vi "OuputMixer5782_1Ghz_interpolated.vi"(8 "input valid":bool=TRUE, 9 "Sine in":fxp<+/-,16,0>[](array[numeric])=[0.0, 0.0, 0.0, 0.0, 0.0, 0.0, 0.0, 0.0], 10 "Cosine in":fxp<+/-,16,0>[](array[numeric])=[0.0, 0.0, 0.0, 0.0, 0.0, 0.0, 0.0, 0.0], 11 "Data":fxp<+/-,16,14>[](array[numeric])=[0.0, 0.0]) -> (3 "test":i16[](array[numeric]))   [LabVIEW 2013]
doc: "Outputs input from channel 0 as I*cos(t)-Q*sin(t) on analog output 0"
uses:
  <vilib>/rvi/eio/common/nirviEmuTemplateMethod_errors.vi
  <vilib>/eio/EIONode/EIONode.xnode
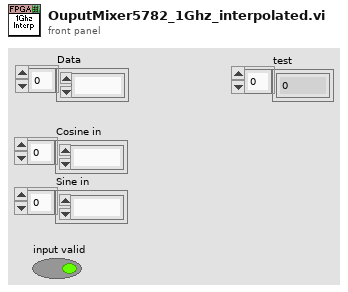
[diagram p1: front panel]
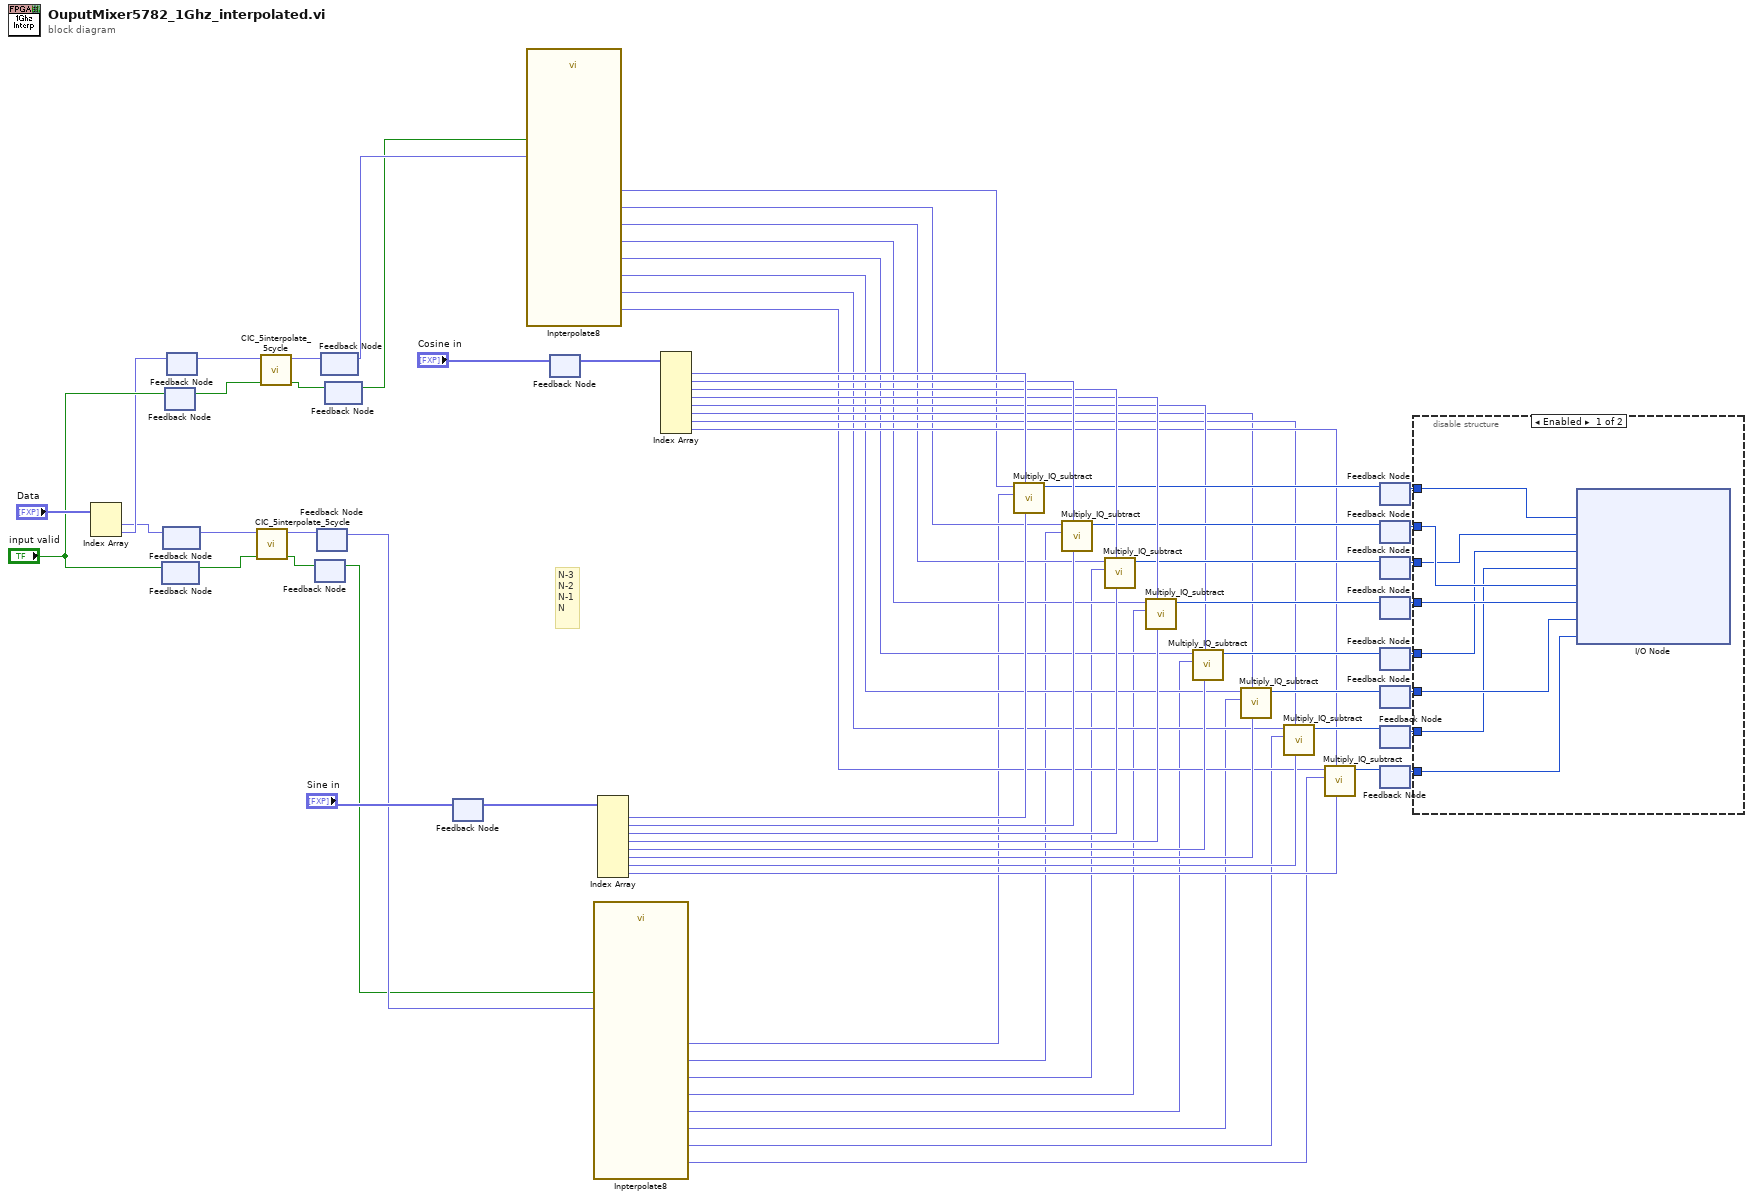
[diagram p0: block diagram]
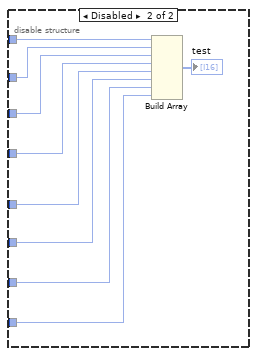
[diagram p2: hidden frame]
diagram:
  # "N-3\nN-2\nN-1\nN"
  n1 = Index Array(array="Data") -> (element #1=w1:fxp<+/-,16,14>, element #2=w2:fxp<+/-,16,14>)  [unwired: 2 in]
  n2 = feedback #1() -> (w13:bool)  [unwired: 1 in]
  n3 = feedback-in #1("input valid") -> ()
  n4 = feedback #2() -> (w15:fxp<+/-,16,14>)  [unwired: 1 in]
  n5 = feedback-in #2(w1) -> ()
  n6 = feedback #3() -> (w14:bool)  [unwired: 1 in]
  n7 = feedback-in #3("input valid") -> ()
  n8 = feedback #4() -> (w16:fxp<+/-,16,14>)  [unwired: 1 in]
  n9 = feedback-in #4(w2) -> ()
  n10 = call "CIC_5interpolate_5cycle.vi"("valid in"=w13, "Data in"=w15) -> ("valid out"=w4:bool, "Data out"=w12:fxp<+/-,16,14>)  [unwired: 8 in]
  n11 = call "CIC_5interpolate_5cycle.vi"("valid in"=w14, "Data in"=w16) -> ("valid out"=w6:bool, "Data out"=w11:fxp<+/-,16,14>)  [unwired: 8 in]
  n12 = feedback #5() -> (w3:bool)  [unwired: 1 in]
  n13 = feedback-in #5(w4) -> ()
  n14 = feedback #6() -> (w7:fxp<+/-,16,14>)  [unwired: 1 in]
  n15 = feedback-in #6(w12) -> ()
  n16 = feedback #7() -> (w8:fxp<+/-,16,14>)  [unwired: 1 in]
  n17 = feedback-in #7(w11) -> ()
  n18 = feedback #8() -> (w5:bool)  [unwired: 1 in]
  n19 = feedback-in #8(w6) -> ()
  n20 = feedback #9() -> (w68:fxp<+/-,16,0>[])  [unwired: 1 in]
  n21 = feedback-in #9("Sine in") -> ()
  n22 = call "Inpterpolate8.vi"("X"=w8, "input valid"=w5) -> ("X(t -7)"=w32:fxp<+/-,16,14>, "X(t -5)"=w30:fxp<+/-,16,14>, "X(t)"=w25:fxp<+/-,16,14>, "X(t -1)"=w26:fxp<+/-,16,14>, "X(t -2)"=w27:fxp<+/-,16,14>, "X(t -3)"=w28:fxp<+/-,16,14>, "X(t -6)"=w31:fxp<+/-,16,14>, "X(t -4)"=w29:fxp<+/-,16,14>)  [unwired: 5 in, 1 out]
  n23 = feedback #10() -> (w67:fxp<+/-,16,0>[])  [unwired: 1 in]
  n24 = feedback-in #10("Cosine in") -> ()
  n25 = call "Inpterpolate8.vi"("X"=w7, "input valid"=w3) -> ("X(t -7)"=w24:fxp<+/-,16,14>, "X(t -5)"=w18:fxp<+/-,16,14>, "X(t)"=w23:fxp<+/-,16,14>, "X(t -1)"=w22:fxp<+/-,16,14>, "X(t -2)"=w21:fxp<+/-,16,14>, "X(t -3)"=w20:fxp<+/-,16,14>, "X(t -6)"=w17:fxp<+/-,16,14>, "X(t -4)"=w19:fxp<+/-,16,14>)  [unwired: 5 in, 1 out]
  n26 = Index Array(array=w68) -> (element #1=w57:fxp<+/-,16,0>, element #2=w58:fxp<+/-,16,0>, element #3=w59:fxp<+/-,16,0>, element #4=w60:fxp<+/-,16,0>, element #5=w51:fxp<+/-,16,0>, element #6=w50:fxp<+/-,16,0>, element #7=w49:fxp<+/-,16,0>, element #8=w48:fxp<+/-,16,0>)  [unwired: 8 in]
  n27 = Index Array(array=w67) -> (element #1=w64:fxp<+/-,16,0>, element #2=w63:fxp<+/-,16,0>, element #3=w62:fxp<+/-,16,0>, element #4=w61:fxp<+/-,16,0>, element #5=w43:fxp<+/-,16,0>, element #6=w40:fxp<+/-,16,0>, element #7=w41:fxp<+/-,16,0>, element #8=w42:fxp<+/-,16,0>)  [unwired: 8 in]
  n28 = call "Multiply_IQ_subtract.vi"("Sin"=w57, "Cos"=w64, "Q"=w24, "I"=w32) -> ("Z"=w56:i16)  [unwired: 6 in, 1 out]
  n29 = call "Multiply_IQ_subtract.vi"("Sin"=w58, "Cos"=w63, "Q"=w17, "I"=w31) -> ("Z"=w55:i16)  [unwired: 6 in, 1 out]
  n30 = call "Multiply_IQ_subtract.vi"("Sin"=w59, "Cos"=w62, "Q"=w18, "I"=w30) -> ("Z"=w54:i16)  [unwired: 6 in, 1 out]
  n31 = call "Multiply_IQ_subtract.vi"("Sin"=w60, "Cos"=w61, "Q"=w19, "I"=w29) -> ("Z"=w53:i16)  [unwired: 6 in, 1 out]
  n32 = call "Multiply_IQ_subtract.vi"("Sin"=w51, "Cos"=w43, "Q"=w20, "I"=w28) -> ("Z"=w47:i16)  [unwired: 6 in, 1 out]
  n33 = call "Multiply_IQ_subtract.vi"("Sin"=w50, "Cos"=w40, "Q"=w21, "I"=w27) -> ("Z"=w46:i16)  [unwired: 6 in, 1 out]
  n34 = call "Multiply_IQ_subtract.vi"("Sin"=w49, "Cos"=w41, "Q"=w22, "I"=w26) -> ("Z"=w45:i16)  [unwired: 6 in, 1 out]
  n35 = call "Multiply_IQ_subtract.vi"("Sin"=w48, "Cos"=w42, "Q"=w23, "I"=w25) -> ("Z"=w44:i16)  [unwired: 6 in, 1 out]
  n36 = feedback #11() -> (w52:i16)  [unwired: 1 in]
  n37 = feedback-in #11(w56) -> ()
  n38 = feedback #12() -> (w39:i16)  [unwired: 1 in]
  n39 = feedback-in #12(w55) -> ()
  n40 = feedback #13() -> (w38:i16)  [unwired: 1 in]
  n41 = feedback-in #13(w54) -> ()
  n42 = feedback #14() -> (w37:i16)  [unwired: 1 in]
  n43 = feedback-in #14(w53) -> ()
  n44 = feedback #15() -> (w36:i16)  [unwired: 1 in]
  n45 = feedback-in #15(w47) -> ()
  n46 = feedback #16() -> (w35:i16)  [unwired: 1 in]
  n47 = feedback-in #16(w46) -> ()
  n48 = feedback #17() -> (w34:i16)  [unwired: 1 in]
  n49 = feedback-in #17(w45) -> ()
  n50 = feedback #18() -> (w33:i16)  [unwired: 1 in]
  n51 = feedback-in #18(w44) -> ()
  n52 = disable-structure shown="Enabled" {
    disable-tunnel: w52 -> [w76 w85]
    disable-tunnel: w39 -> [w75 w84]
    disable-tunnel: w38 -> [w74 w83]
    disable-tunnel: w37 -> [w73 w82]
    disable-tunnel: w36 -> [w72 w81]
    disable-tunnel: w35 -> [w71 w80]
    disable-tunnel: w34 -> [w70 w79]
    disable-tunnel: w33 -> [w69 w78]
    frame Enabled {
      n53 = xnode "I/O Node"("IO Module\\AO 0 N-3"=w76, "IO Module\\AO 0 N-2"=w74, "IO Module\\AO 0 N-1"=w72, "IO Module\\AO 0 N"=w70, "IO Module\\AO 1 N-3"=w75, "IO Module\\AO 1 N-2"=w73, "IO Module\\AO 1 N-1"=w71, "IO Module\\AO 1 N"=w69) -> ()  [unwired: 8 in, 8 out]
    }
    frame Disabled {
      n54 = Build Array(w85, w84, w83, w82, w81, w80, w79, w78) -> (→"test":i16[])
    }
  }
